vi "Convert Java Time.vi"(11 "Date/Time":string) -> (3 "Time Stamp":timestamp)   [LabVIEW 2011]
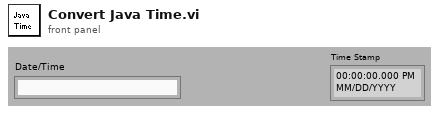
[diagram p1: front panel]
types:
  T1 = cluster{"second":i32, "minute":i32, "hour":i32, "day of month":i32, "month":i32, "year":i32, "day of week":i32, "day of year":i32, "is DST":i32}
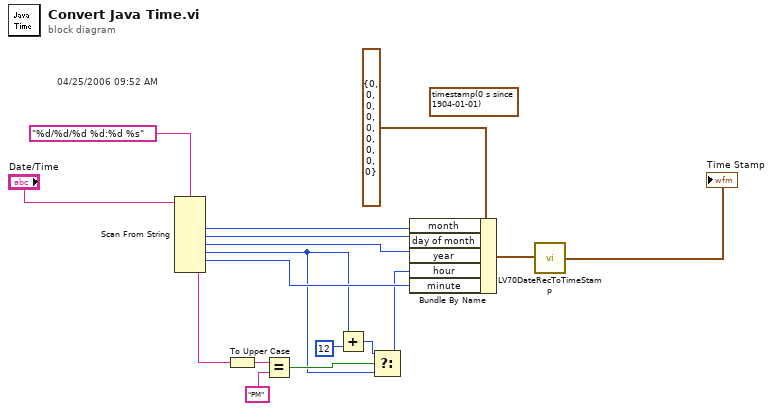
[diagram p0: block diagram]
diagram:
  (unwired) timestamp(0 s since 1904-01-01) ("Time Stamp")
  # "04/25/2006 09:52 AM"
  n1 = Scan From String(format string="%d/%d/%d %d:%d %s" ("string"), input string="Date/Time") -> (output 1=w12:i32, output 2=w11:i32, output 3=w10:i32, output 4=w3:i32, output 5=w9:i32, output 6=w6:string)  [unwired: 2 in, 9 out]
  n2 = To Upper Case(1:w6) -> (0:w7:string)
  n3 = Equal?(x=w7, y="PM" ("string")) -> (x = y?=w5:bool)
  n4 = Add(x=w3, y=12) -> (x+y=w4:i32)
  n5 = Select(t=w4, s=w5, f=w3) -> (s? t:f=w2:i32)
  n6 = Bundle By Name(cluster=T1 {"second"=0, "minute"=0, "hour"=0, "day of month"=0, "month"=0, "year"=0, "day of week"=0, "day of year"=0, "is DST"=0} ("date time rec"), "month"=w12, "day of month"=w11, "year"=w10, "hour"=w2, "minute"=w9) -> (w14:T1)
  n7 = call <vilib>:"LV70DateRecToTimeStamp.vi"("date time rec"=w14) -> ("Time Stamp"=→"Time Stamp":timestamp)
